vi "Create Channel.vi"(6 "New Section Name (none)":string, 8 "error in":errorcluster, 9 "Type":T2, 10 "Channel":T1, 11 "Item Ref in":T3 format="%.0x") -> (0 "error out":errorcluster, 3 "Item Ref out":T3 format="%.0x")   [LabVIEW 2017, in "PXImc System Explorer.lvlib"]
uses:
  PXImc System Explorer.lvlib
  <vilib>/NI Veristand/Custom Device API/Custom Device Item Ref.ctl
  <vilib>/NI Veristand/Custom Device API/Custom Device Channel Type.ctl
  Shared/Channel.ctl
  <vilib>/NI Veristand/Custom Device API/Custom Device Channel.ctl
  Shared/Constants.vi
  <vilib>/NI VeriStand/Custom Device API/Custom Device API.lvlib
  Shared/PXImc Shared.lvlib
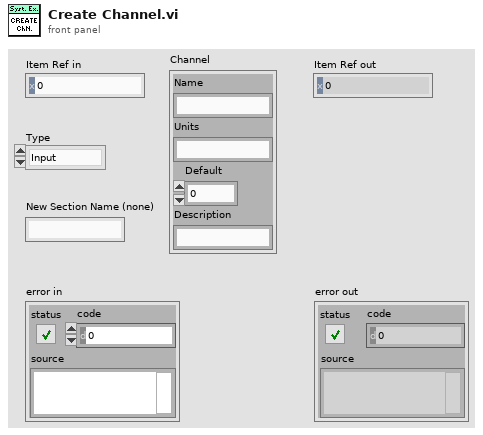
[diagram p1: front panel]
types:
  T1 = typedef "PXImc Shared.lvlib/Channel.ctl" = cluster{"Name":string, "Units":string, "Default":dbl, "Description":string}
  T2 = typedef "Custom Device API.lvlib/Custom Device Channel Type.ctl" = enum16{"Input", "Output"}
  T3 = typedef "Custom Device API.lvlib/Custom Device Item Ref.ctl" = u64
  T4 = typedef "Custom Device API.lvlib/Custom Device Channel.ctl" = cluster{"Type":T2, "Units":string, "Default Value":dbl, "Faultable":bool, "Scalable":bool}
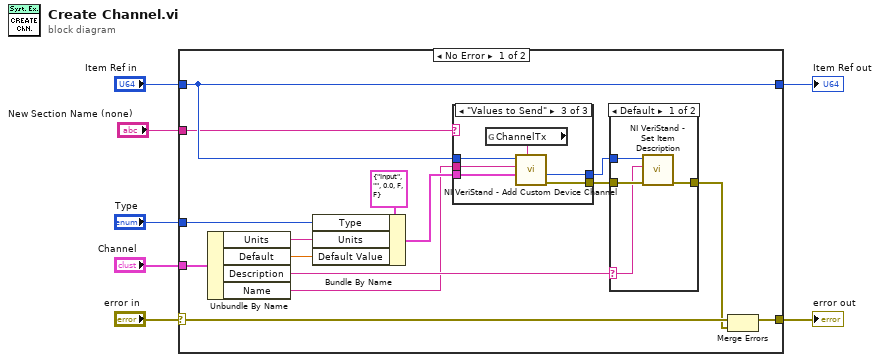
[diagram p0: block diagram]
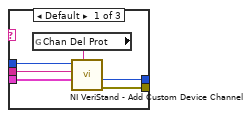
[diagram p2: hidden frame]
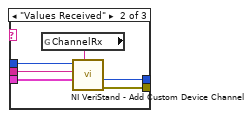
[diagram p3: hidden frame]
diagram:
  n1 = case shown="No Error" "error in" {
    selector: "error in" -> [w22 w46]
    tunnel: [w21 w46] -> w6
    tunnel: [w9 w47] -> w5
    tunnel: "Item Ref in" -> [w9 w47]
    tunnel: "Type" -> [w10 _]
    tunnel: "Channel" -> [w11 _]
    tunnel: "New Section Name (none)" -> [w8 _]
    frame No Error {
      n2 = Unbundle By Name(w11) -> ("Units"=w17:string, "Default"=w16:dbl, "Description"=w15:string, "Name"=w13:string)
      n3 = Bundle By Name(cluster=T4 {"Type"=enum."Input", "Units"="", "Default Value"=0.0, "Faultable"=FALSE, "Scalable"=FALSE} ("Channel"), "Type"=w10, "Units"=w17, "Default Value"=w16) -> (w20:T4)
      n4 = case shown="\"Values to Send\"" w8 {
        tunnel: w20 -> [w28 w34 w40]
        tunnel: [w27 w33 w39] -> w19
        tunnel: [w26 w32 w38] -> w18
        tunnel: w9 -> [w24 w30 w36]
        tunnel: w13 -> [w23 w29 w35]
        frame Default {
          n5 = global read "Constants.vi" "Chan Del Prot"() -> (w25:string)
          n6 = call <vilib>:"NI VeriStand - Add Custom Device Channel.vi"("GUID (Default Channel)"=w25, "Channel"=w28, "Channel Name"=w23, "Parent Ref in"=w24) -> ("error out"=w27:errorcluster, "Channel Ref"=w26:T3)  [unwired: 4 in, 2 out]
        }
        frame "Values Received" {
          n7 = global read "Constants.vi" "ChannelRx"() -> (w31:string)
          n8 = call <vilib>:"NI VeriStand - Add Custom Device Channel.vi"("GUID (Default Channel)"=w31, "Channel"=w34, "Channel Name"=w29, "Parent Ref in"=w30) -> ("error out"=w33:errorcluster, "Channel Ref"=w32:T3)  [unwired: 4 in, 2 out]
        }
        frame "Values to Send" {
          n9 = global read "Constants.vi" "ChannelTx"() -> (w37:string)
          n10 = call <vilib>:"NI VeriStand - Add Custom Device Channel.vi"("GUID (Default Channel)"=w37, "Channel"=w40, "Channel Name"=w35, "Parent Ref in"=w36) -> ("error out"=w39:errorcluster, "Channel Ref"=w38:T3)  [unwired: 4 in, 2 out]
        }
      }
      n11 = case shown="Default" w15 {
        selector: w15 -> [w41 _]
        tunnel: [w43 w45] -> w12
        tunnel: w19 -> [w44 w45]
        tunnel: w18 -> [w42 _]
        frame Default {
          n12 = call <vilib>:"NI VeriStand - Set Item Description.vi"("error in (no error)"=w44, "Description"=w41, "Item Ref in"=w42) -> ("error out"=w43:errorcluster)  [unwired: 6 in, 2 out]
        }
        frame "" {
        }
      }
      n13 = Merge Errors(w22, w12) -> (w21:errorcluster)
    }
    frame Error {
    }
  }
  "error out" <- w6
  "Item Ref out" <- w5
